vi "PPR_DRIVE_Get_WheelDistances.vi"() -> (1 "Right Wheel Dist M":dbl format="%17.2f", 3 "Left Wheel Dist M":dbl format="%17.2f")   [LabVIEW 2019]
uses:
  PPR_DRIVE_GLOBALS.vi
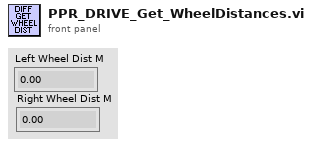
[diagram p1: front panel]
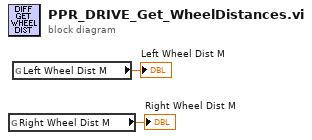
[diagram p0: block diagram]
diagram:
  n1 = global read "PPR_DRIVE_GLOBALS.vi" "Right Wheel Dist M"() -> (→"Right Wheel Dist M":dbl)
  n2 = global read "PPR_DRIVE_GLOBALS.vi" "Left Wheel Dist M"() -> (→"Left Wheel Dist M":dbl)
